vi "SetClassQueueMessage.vi"(8 "ErrorIn(No Error)":errorcluster caption="entrée d'erreur (pas d'erreur)", 10 "Menu déroulant":T1 items=["UpdateClassData", "UpdateMainClass"], 11 "OR77200.lvclass":refnum<class "OR77200.lvclass">) -> (0 "sortie d'erreur":errorcluster, 3 "OR77200.lvclass Out":refnum<class "OR77200.lvclass">)   [LabVIEW 2019, in "OR77200.lvclass"]
uses:
  OR77200.lvclass
  BaseDevice/ClassQueueMess.ctl
  BaseDevice/BaseDevice.lvclass
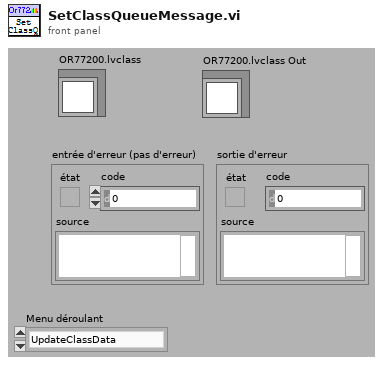
[diagram p1: front panel]
types:
  T1 = typedef "ClassQueueMess.ctl" = u16
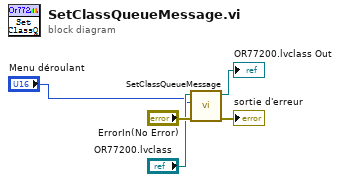
[diagram p0: block diagram]
diagram:
  n1 = call-parent "SetClassQueueMessage.vi"("ErrorIn(No Error)"="ErrorIn(No Error)", "Menu déroulant"="Menu déroulant", "BaseDevice.lvclass"="OR77200.lvclass") -> ("sortie d'erreur"=→"sortie d'erreur":errorcluster, "BaseDevice.lvclass Out"=→"OR77200.lvclass Out":refnum<class "OR77200.lvclass">)  [unwired: 7 in]
